vi "_tester_.vi"() -> ()   [LabVIEW 2025]
uses:
  LabVIEWpcm.dll
panel:
  out "Waveform Chart 4":u64(graph)
  out "Waveform Chart 3":dbl(graph)
  out "Waveform Chart 2":u64(graph)
  out "Waveform Chart":dbl(graph)
  in  "Stop Button":bool
  out "l3miss":u64
  out "l3hit":dbl
  out "lv2miss":u64
  out "lv2hit":dbl
  out "init":i32
  out "return type":i32
  out "bytes":u64
  out "ipc":dbl
  # "MUST BE RUN AS ADMINISTRATOR!!!"
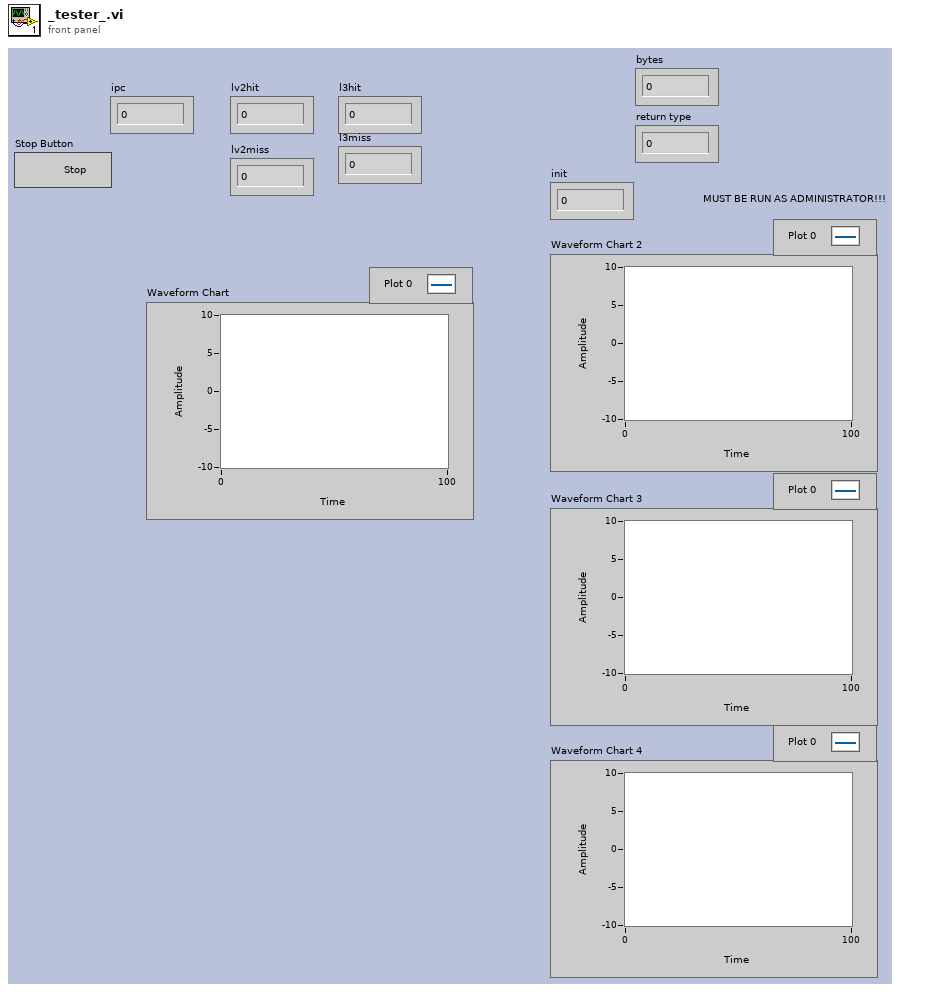
[diagram p1: front panel]
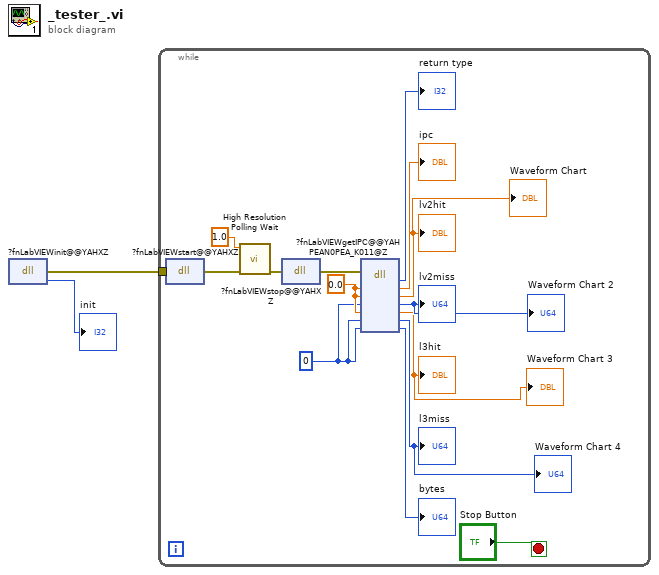
[diagram p0: block diagram]
diagram:
  n1 = dll-call lib="C:/Users/Andrey/Desktop/intel-pcm/build/x64/Release/LabVIEWpcm.dll" fn="?fnLabVIEWinit@@YAHXZ"() -> (error out=w2:errorcluster, "return type"=→"init":i32)  [unwired: 3 in, 1 out]
  n2 = while {
    tunnel: w2 -> [w17]
    stop <- "Stop Button" stop-if-true
    w8 = u64 0 ("bytes")
    w9 = 0.0 ("ipc")
    n3 = dll-call lib="C:/Users/Andrey/Desktop/intel-pcm/build/x64/Release/LabVIEWpcm.dll" fn="?fnLabVIEWstart@@YAHXZ"(error in=w17) -> (error out=w16:errorcluster)  [unwired: 3 in, 1 out]
    n4 = call <vilib>:"High Resolution Polling Wait.vi"("error in (no error)"=w16, "seconds to wait"=1.0) -> ("error out"=w15:errorcluster)  [unwired: 9 in]
    n5 = dll-call lib="C:/Users/Andrey/Desktop/intel-pcm/build/x64/Release/LabVIEWpcm.dll" fn="?fnLabVIEWstop@@YAHXZ"(error in=w15) -> (error out=w14:errorcluster)  [unwired: 3 in, 1 out]
    n6 = dll-call lib="C:/Users/Andrey/Desktop/intel-pcm/build/x64/Release/LabVIEWpcm.dll" fn="?fnLabVIEWgetIPC@@YAHPEAN0PEA_K011@Z"(error in=w14, "ipc"=w9, "lv2hit"=w9, "lv2miss"=w8, "l3hit"=w9, "l3miss"=w8, "bytes"=w8) -> ("return type"=→"return type":i32, "ipc"=→"ipc":dbl, "lv2hit"=→"lv2hit" →"Waveform Chart":dbl, "lv2miss"=→"lv2miss" →"Waveform Chart 2":u64, "l3hit"=→"l3hit" →"Waveform Chart 3":dbl, "l3miss"=→"l3miss" →"Waveform Chart 4":u64, "bytes"=→"bytes":u64)  [unwired: 2 in, 2 out]
  }
